vi "1259_usbUart.vi"(0 "VISA resource name":refnum<visa-resource-name>, 1 "write buffer":string, 2 "sdFeature":bool, 5 "error in (no error)":errorcluster) -> (3 "byte integer string":string[](array[string]), 4 "double precision float":dbl, 6 "binary[0] String":string, 7 "binary[1] String":string, 8 "byte[0]":string, 9 "maxSpeed":string, 10 "read buffer":string, 11 "BB FW":string, 12 "valid byte":string, 13 "PartNumber":string, 14 "number[0]":u32, 15 "number[1]":u32, 16 "number[2]":u32, 17 "number[3]":u32, 18 "negative incline":dbl, 19 "error out":errorcluster)   [LabVIEW 2018]
uses:
  <vilib>/Instr/_visa.llb/VISA Flush IO Buffer Mask.ctl
  <vilib>/Instr/_visa.llb/VISA Configure Serial Port (Instr).vi
panel:
  out "filterString":string
  out "length":i32
  out "bytes [0, 1]":string
  out "byte[3]":string
  out "DMK":string
  out "USB":string
  out "binary[2] String":string
  out "bytes [0, 1, 2]":string
  out "byte[2]":string
  out "TV":string
  out "DEMO":string
  out "WAHOO":string
  out "CSAFE":string
  out "TABLET":string
  out "PULSE":string
  out "RESISTANCE":string
  out "BLE":string
  out "byte[1] array":string[](array[string])
  out "BUZZER":string
  out "AUDIO":string
  out "FAN":string
  out "DISTANCE":string
  out "GRADE":string
  out "SPEED":string
  out "byte[0] array":string[](array[string])
  out "byte[1]":string
  out "bytes at port":u32
  out "byte count":u32
  # "BYTE[0] AND BYTE[1] ARE GENERAL PURPOSE AND FEATURE PARSING"
  # "BYTE[3] NEEDED FOR BRAINBOARD FIRMWARE"
  # "BYTE[2] NEEDED FOR PART NUMBER"
  # "BYTE[0] AND BYTE[1] SWAPPED FOR MAX SPEED ONLY"
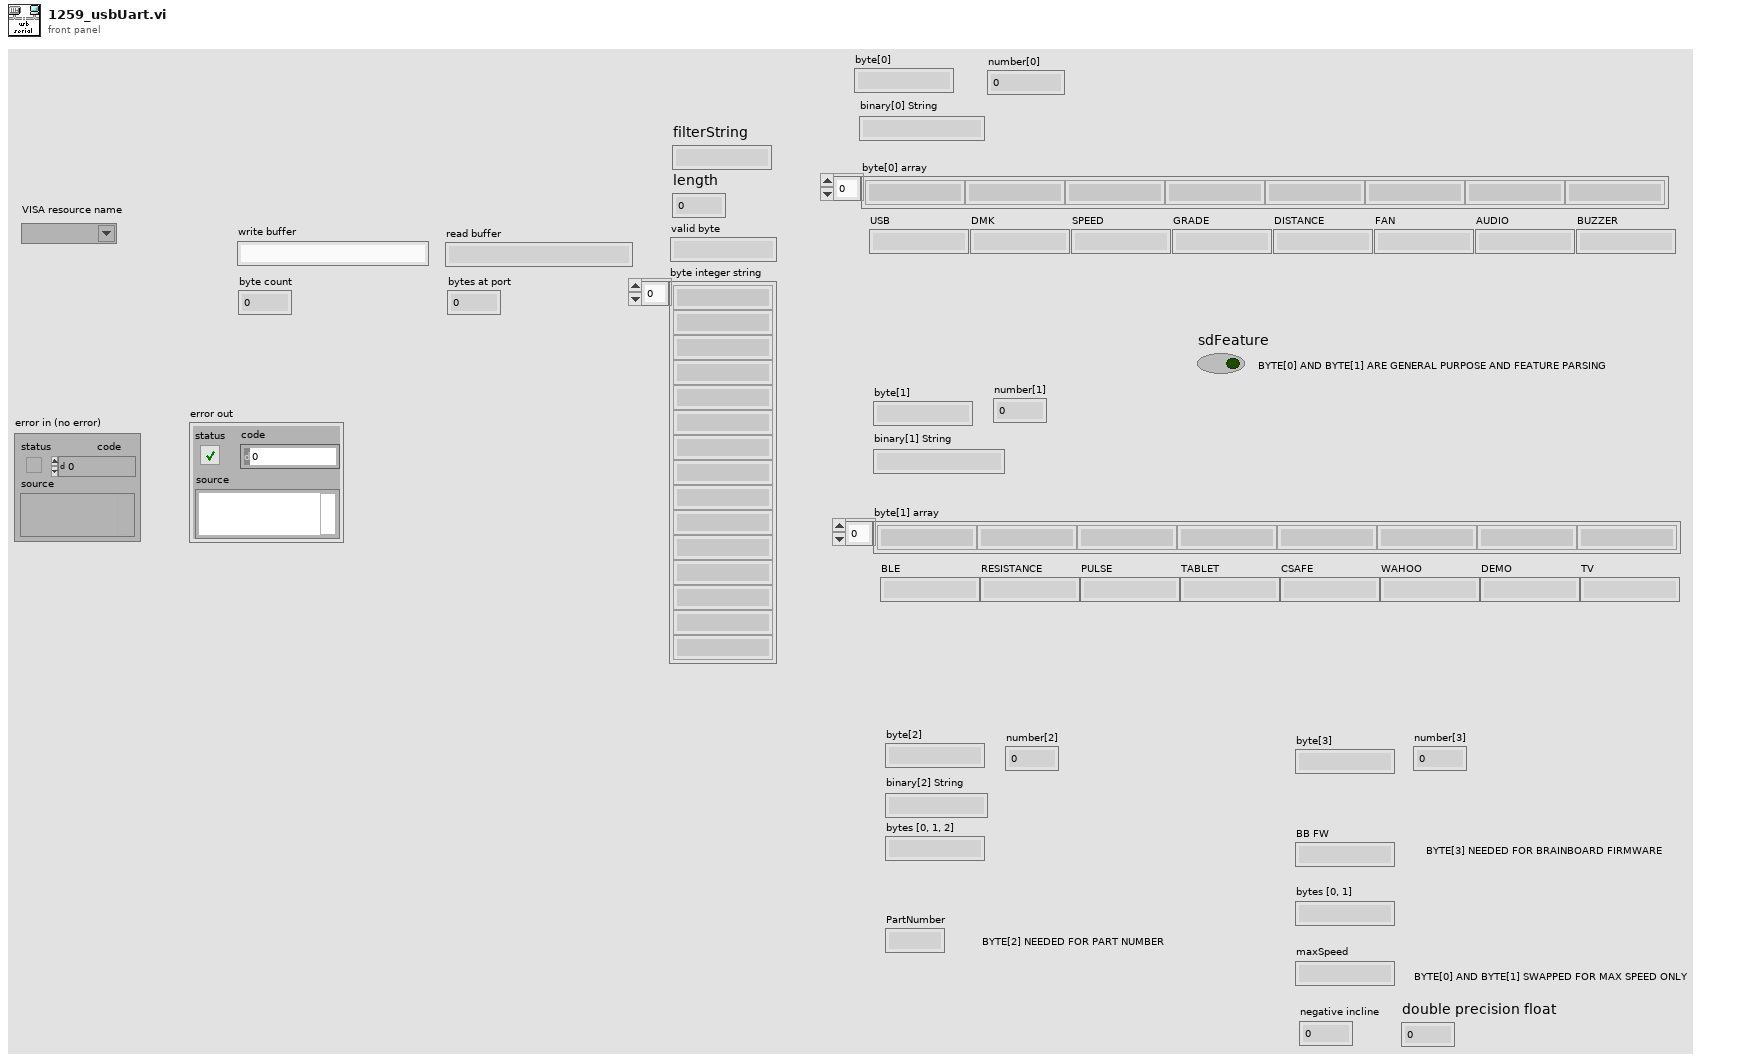
[diagram p1: front panel]
types:
  T1 = typedef "VISA Flush IO Buffer Mask.ctl" = u16
  T2 = cluster{"[0]":string, "[1]":string, "[2]":string, "[3]":string, "[4]":string, "[5]":string, "[6]":string, "[7]":string, "[8]":string}
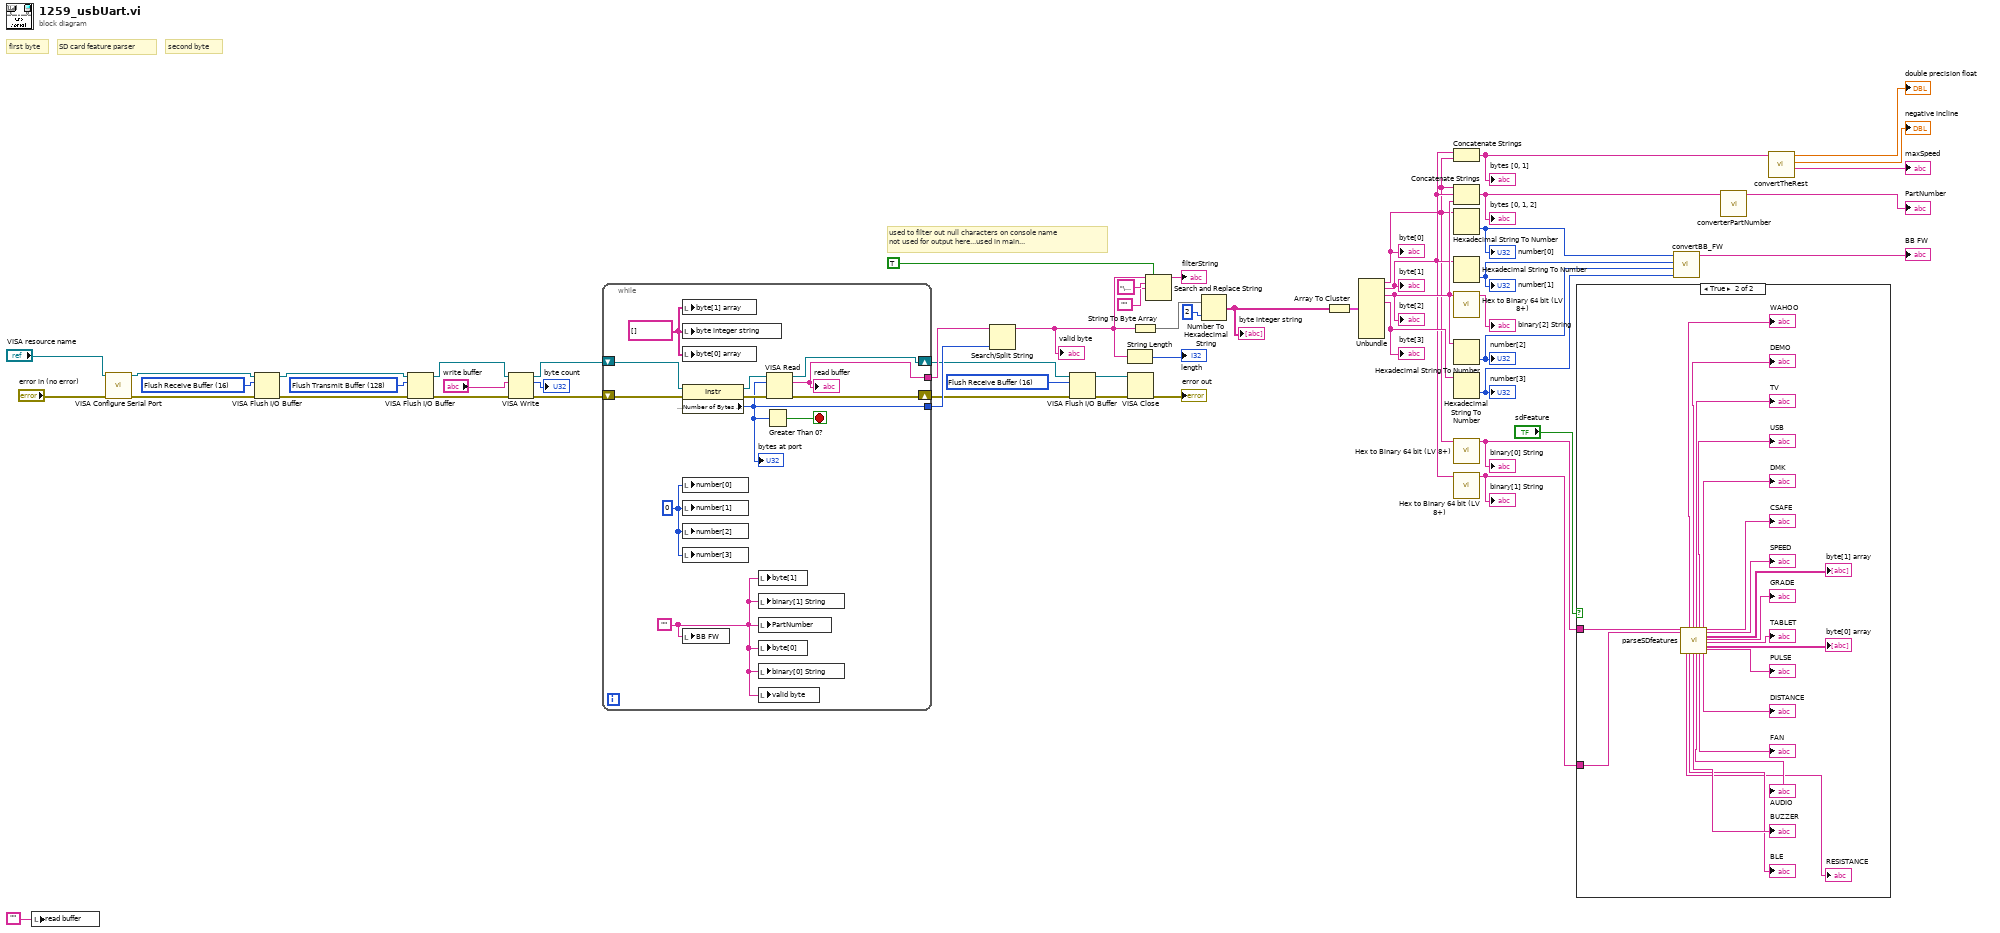
[diagram p0: block diagram]
diagram:
  w32 = T1 128 items=["Flush Receive Buffer"=16, "Write Transmit Buffer to Device"=32, "Flush Receive Buffer (No I/O)"=64, "Flush Transmit Buffer"=128] ("Mask")
  w36 = T1 16 items=["Flush Receive Buffer"=16, "Write Transmit Buffer to Device"=32, "Flush Receive Buffer (No I/O)"=64, "Flush Transmit Buffer"=128] ("Mask")
  w39 = T1 16 items=["Flush Receive Buffer"=16, "Write Transmit Buffer to Device"=32, "Flush Receive Buffer (No I/O)"=64, "Flush Transmit Buffer"=128] ("Mask")
  # "used to filter out null characters on console name\nnot used for output here...used in main..."
  # "second byte"
  # "first byte"
  # "SD card feature parser"
  n1 = local write "read buffer"("") -> ()
  n2 = call-poly "VISA Configure Serial Port"("VISA resource name"="VISA resource name", "error in (no error)"="error in (no error)") -> ("VISA resource name out"=w38:refnum<visa-resource-name>, "error out"=w37:errorcluster)  [unwired: 12 in]
  n3 = VISA Flush I/O Buffer(VISA resource name=w38, mask (16)=w36, error in (no error)=w37) -> (VISA resource name out=w33:refnum<visa-resource-name>, error out=w34:errorcluster)
  n4 = VISA Flush I/O Buffer(VISA resource name=w33, mask (16)=w32, error in (no error)=w34) -> (VISA resource name out=w31:refnum<visa-resource-name>, error out=w30:errorcluster)
  n5 = VISA Write(VISA resource name=w31, write buffer="write buffer", error in (no error)=w30) -> (VISA resource name out=w52:refnum<visa-resource-name>, return count=→"byte count":u32, error out=w51:errorcluster)
  n6 = while {
    tunnel: [w57] -> w49
    tunnel: [w59] -> w45
    shift-right: [w54] -> w35
    shift-left: w52 -> [w64]
    shift-right: [w55] -> w40
    shift-left: w51 -> [w63]
    stop <- w60 stop-if-true
    w56 = u32 0
    w58 = string[] []
    w53 = ""
    n7 = local write "byte[1] array"(w58) -> ()
    n8 = local write "byte integer string"(w58) -> ()
    n9 = local write "byte[0] array"(w58) -> ()
    n10 = property class="Instr"(reference=w64, error in=w63) -> (reference out=w61:refnum<visa-resource-name>, error out=w62:errorcluster, "Serial Settings:Number of Bytes at Serial Port"=w59:u32)
    "bytes at port" <- w59
    n11 = local write "number[0]"(w56) -> ()
    n12 = local write "number[1]"(w56) -> ()
    n13 = local write "number[2]"(w56) -> ()
    n14 = local write "number[3]"(w56) -> ()
    n15 = local write "BB FW"(w53) -> ()
    n16 = local write "byte[1]"(w53) -> ()
    n17 = local write "binary[1] String"(w53) -> ()
    n18 = local write "PartNumber"(w53) -> ()
    n19 = local write "byte[0]"(w53) -> ()
    n20 = local write "binary[0] String"(w53) -> ()
    n21 = local write "valid byte"(w53) -> ()
    n22 = Greater Than 0?(x=w59) -> (x > 0?=w60:bool)
    n23 = VISA Read(VISA resource name=w61, byte count=w59, error in (no error)=w62) -> (VISA resource name out=w54:refnum<visa-resource-name>, read buffer=w57:string, error out=w55:errorcluster)  [unwired: 1 out]
    "read buffer" <- w57
  }
  n24 = Search/Split String(string=w49, offset (0)=w45) -> (substring before match=w21:string)  [unwired: 1 in, 2 out]
  "valid byte" <- w21
  n25 = VISA Flush I/O Buffer(VISA resource name=w35, mask (16)=w39, error in (no error)=w40) -> (VISA resource name out=w29:refnum<visa-resource-name>, error out=w28:errorcluster)
  n26 = String Length(string=w21) -> (length=→"length":i32)
  n27 = VISA Close(VISA resource name=w29, error in (no error)=w28) -> (error out=→"error out":errorcluster)
  n28 = String To Byte Array(string=w21) -> (unsigned byte array=w48:u8[])
  n29 = Search and Replace String(replace all?=TRUE ("replace all? (F)"), input string=w21, search string="\u0000", replace string="") -> (result string=→"filterString":string)  [unwired: 4 in, 3 out]
  n30 = Number To Hexadecimal String(1:i16 2 ("width (-)"), 2:w48) -> (0:w47:string[])
  "byte integer string" <- w47
  n31 = Array To Cluster(array=w47) -> (cluster=w46:T2)
  n32 = Unbundle(w46) -> ("[0]"=w1:string, "[1]"=w2:string, "[2]"=w42:string, "[3]"=w41:string)  [unwired: 5 out]
  "byte[0]" <- w1
  "byte[1]" <- w2
  "byte[2]" <- w42
  "byte[3]" <- w41
  n33 = Concatenate Strings(w2, w1) -> (w4:string)
  "bytes [0, 1]" <- w4
  n34 = Concatenate Strings(w1, w2, w42) -> (w14:string)
  "bytes [0, 1, 2]" <- w14
  n35 = Hexadecimal String To Number(string=w1) -> (number=w13:u32)  [unwired: 2 in, 1 out]
  "number[0]" <- w13
  n36 = Hexadecimal String To Number(string=w2) -> (number=w12:u32)  [unwired: 2 in, 1 out]
  "number[1]" <- w12
  n37 = call "Hex to Binary 64 bit (LV 8+).vi"("Hexadecimal String"=w42) -> ("Binary String"=→"binary[2] String":string)  [unwired: 6 in, 2 out]
  n38 = Hexadecimal String To Number(string=w42) -> (number=w11:u32)  [unwired: 2 in, 1 out]
  "number[2]" <- w11
  n39 = Hexadecimal String To Number(string=w41) -> (number=w10:u32)  [unwired: 2 in, 1 out]
  "number[3]" <- w10
  n40 = call "Hex to Binary 64 bit (LV 8+).vi"("Hexadecimal String"=w1) -> ("Binary String"=w9:string)  [unwired: 6 in, 2 out]
  "binary[0] String" <- w9
  n41 = call "Hex to Binary 64 bit (LV 8+).vi"("Hexadecimal String"=w2) -> ("Binary String"=w8:string)  [unwired: 6 in, 2 out]
  "binary[1] String" <- w8
  n42 = case shown="True" "sdFeature" {
    tunnel: w9 -> [_ w66]
    tunnel: w8 -> [_ w65]
    frame False {
    }
    frame True {
      n43 = call "parseSDfeatures.vi"("binary[0] string"=w66, "binary[1] string"=w65) -> ("RESISTANCE"=→"RESISTANCE":string, "WAHOO"=→"WAHOO":string, "BLE"=→"BLE":string, "DEMO"=→"DEMO":string, "BUZZER"=→"BUZZER":string, "TV"=→"TV":string, "AUDIO"=→"AUDIO":string, "USB"=→"USB":string, "FAN"=→"FAN":string, "DMK"=→"DMK":string, "DISTANCE"=→"DISTANCE":string, "CSAFE"=→"CSAFE":string, "SPEED"=→"SPEED":string, "byte[1] array"=→"byte[1] array":string[], "GRADE"=→"GRADE":string, "TABLET"=→"TABLET":string, "byte[0] array"=→"byte[0] array":string[], "PULSE"=→"PULSE":string)  [unwired: 8 in]
    }
  }
  n44 = call "convertBB_FW.vi"("Numeric [3]"=w10, "Numeric [2]"=w11, "Numeric [1]"=w12, "Numeric [0]"=w13) -> ("BB FW"=→"BB FW":string)  [unwired: 7 in]
  n45 = call "converterPartNumber.vi"("bytes [0, 1, 2]"=w14) -> ("PartNumber"=→"PartNumber":string)  [unwired: 10 in]
  n46 = call "convertTheRest.vi"("byte [0, 1]"=w4) -> ("maxSpeed"=→"maxSpeed":string, "negative incline"=→"negative incline":dbl, "double precision float"=→"double precision float":dbl)  [unwired: 8 in]
